vi "main(Test DQMH modules).vi"() -> ()   [LabVIEW 2018, in "Application.lvlib"] (continued)
        n826 = call "Connect to CE14.vi"("Module ID"=-1) -> ("error out"=w1953:errorcluster)  [unwired: 10 in]
        n827 = Merge Errors(w1949, w1953) -> (w1946:errorcluster)
        n828 = flat-sequence {
          tunnel: [w1959] -> w1947
          tunnel: w1946 -> [w1959]
          frame #0 {
            n829 = Wait (ms)(milliseconds to wait=u32 70) -> ()  [unwired: 1 out]
          }
        }
      }
      frame "MEAS.Read EMIC connected" {
        n830 = disable-structure shown="LOGGING==TRUE" {
          disable-tunnel: w1981 -> [w1999 _]
          frame condition #0 (active) {
            n831 = Empty String/Path?(string/path=w1999) -> (empty?=w2002:bool)
            n832 = Select(t="Quece timeout", s=w2002, f=w1999) -> (s? t:f=w1998:string)
            n833 = call "string log (SubVI).vi"("Enum"=enum16{"Init", "Log", "Read"}."Log", "state Name"=w1998) -> ()  [unwired: 8 in, 2 out]
          }
          frame condition #1 {
          }
        }
        n834 = local read "CE14  Module did it"() -> (w1967:bool[])
        n835 = for {
          N: 6 -> [_]
          tunnel: [w2005] -> w1980 mode=indexing
          tunnel: [w2004] -> w1985 mode=indexing
          i -> [w2007]
          n836 = Increment(x=w2007) -> (x+1=w2006:i32)
          n837 = Wait (ms)(milliseconds to wait=u32 50) -> ()  [unwired: 1 out]
          n838 = call "CE14.CheckConnected.vi"("Module ID"=w2006) -> ("error out"=w2004:errorcluster, "Success"=w2005:bool)  [unwired: 8 in, 1 out]
        }
        "EMIC connected" <- w1980
        n839 = And(x=w1967, y=w1980) -> (x .and. y?=w1970:bool[])
        n840 = Index Array(array=w1970) -> (element #1=→"Inst. 4":bool, element #2=→"Inst. 5":bool, element #3=→"Inst. 6":bool, element #4=→"Inst. 7":bool, element #5=→"Inst. 8":bool, element #6=→"Inst. 9":bool)  [unwired: 6 in]
        n841 = Merge Errors(w1984, w1985) -> (w1972:errorcluster)
        n842 = for {
          tunnel: w1970 -> [w1995] mode=indexing
          tunnel: [w1994] -> w1969
          n843 = call "FGV Init phase.vi"("Boolean"=w1995) -> ("Init Completed?"=w1994:bool)  [unwired: 9 in, 1 out]
        }
        n844 = case shown="False" w1969 {
          tunnel: w1968 -> [_ w1993]
          tunnel: [_ w1991] -> w1965
          frame False {
          }
          frame True {
            n845 = call "App enquece.vi"("command"="INIT.Read DRV code", "queue in"=w1993) -> ("error out"=w1991:errorcluster)  [unwired: 8 in, 1 out]
          }
        }
        n846 = Merge Errors(w1972, w1965) -> (w1966:errorcluster)
        n847 = flat-sequence {
          tunnel: [w1996] -> w1973
          tunnel: w1966 -> [w1996]
          frame #0 {
            n848 = Wait (ms)(milliseconds to wait=u32 70) -> ()  [unwired: 1 out]
          }
        }
      }
      frame "MEAS.Set DMM config" {
        n849 = disable-structure shown="LOGGING==TRUE" {
          disable-tunnel: w2011 -> [w2030 _]
          frame condition #0 (active) {
            n850 = Empty String/Path?(string/path=w2030) -> (empty?=w2033:bool)
            n851 = Select(t="Quece timeout", s=w2033, f=w2030) -> (s? t:f=w2029:string)
            n852 = call "string log (SubVI).vi"("Enum"=enum16{"Init", "Log", "Read"}."Log", "state Name"=w2029) -> ()  [unwired: 8 in, 2 out]
          }
          frame condition #1 {
          }
        }
        n853 = Variant To Data(type=T19 {"DMM config cluster"={"DCV range"=0.0, "DCI range"=0.0, "Detector Rate"=0}, "mux2-1(DMM I) encode"=enum."DMM I (0.5)"} ("DMM all config"), Variant=w2023) -> (data=w2021:T19)  [unwired: 1 in, 1 out]
        n854 = Unbundle By Name(w2021) -> ("DMM config cluster"=w2020:T20)
        n855 = Unbundle By Name(w2020) -> ("DCV range"=w2019:dbl, "DCI range"=w2018:dbl, "Detector Rate"=w2017:u8)
        n856 = call "config channel.vi"("Detector Rate"=w2017, "DCI range"=w2018, "DCV range"=w2019) -> ("error out"=w2015:errorcluster)  [unwired: 8 in]
        n857 = Merge Errors(w2012, w2015) -> (w2009:errorcluster)
        n858 = flat-sequence {
          tunnel: [w2028] -> w2010
          tunnel: w2009 -> [w2028]
          frame #0 {
            n859 = Wait (ms)(milliseconds to wait=u32 70) -> ()  [unwired: 1 out]
          }
        }
      }
      frame "MEAS.AllRelaysOFF" {
        n860 = disable-structure shown="LOGGING==TRUE" {
          disable-tunnel: w2036 -> [w2047 _]
          frame condition #0 (active) {
            n861 = Empty String/Path?(string/path=w2047) -> (empty?=w2050:bool)
            n862 = Select(t="Quece timeout", s=w2050, f=w2047) -> (s? t:f=w2046:string)
            n863 = call "string log (SubVI).vi"("Enum"=enum16{"Init", "Log", "Read"}."Log", "state Name"=w2046) -> ()  [unwired: 8 in, 2 out]
          }
          frame condition #1 {
          }
        }
        n864 = for {
          N: 5 -> [_]
          tunnel: [w2051] -> w2041 mode=indexing
          i -> [w2053]
          n865 = case shown="4" w2053 {
            tunnel: [w2057 w2058 w2059 w2060 w2061 _] -> w2051
            frame 0 {
              n866 = Initialize Array(FALSE, 6 ("dimension size")) -> (w2054:bool[])
              n867 = call "MB01_eMICs.vi"("Array"=w2054) -> ("error out"=w2057:errorcluster)  [unwired: 10 in]
            }
            frame 1 {
              n868 = call "demux1-10_chan0.vi"() -> ("error out"=w2058:errorcluster)  [unwired: 11 in]
            }
            frame 2 {
              n869 = call "SC enable OFF.vi"() -> ("error out"=w2059:errorcluster)  [unwired: 11 in]
            }
            frame 3 {
              n870 = call "mux10-1_chan0.vi"() -> ("error out"=w2060:errorcluster)  [unwired: 11 in]
            }
            frame 4 {
              n871 = call "mux6-1_chan0.vi"() -> ("error out"=w2061:errorcluster)  [unwired: 11 in]
            }
            frame 5.., Default {
            }
          }
          n872 = Wait (ms)(milliseconds to wait=u32 70) -> ()  [unwired: 1 out]
        }
        n873 = Merge Errors(w2037, w2041) -> (w2034:errorcluster)
      }
      frame "MEAS.AllRelaysOFF2" {
        # "Turn eMICs' relays OFF"
        n874 = disable-structure shown="LOGGING==TRUE" {
          disable-tunnel: w2065 -> [w2079 _]
          frame condition #0 (active) {
            n875 = Empty String/Path?(string/path=w2079) -> (empty?=w2082:bool)
            n876 = Select(t="Quece timeout", s=w2082, f=w2079) -> (s? t:f=w2078:string)
            n877 = call "string log (SubVI).vi"("Enum"=enum16{"Init", "Log", "Read"}."Log", "state Name"=w2078) -> ()  [unwired: 8 in, 2 out]
          }
          frame condition #1 {
          }
        }
        n878 = flat-sequence {
          tunnel: [w2077] -> w2063
          frame #0 {
            n879 = Initialize Array(FALSE, 6 ("dimension size")) -> (w2076:bool[])
            n880 = Wait (ms)(milliseconds to wait=u32 70) -> ()  [unwired: 1 out]
            n881 = call "MB01_eMICs.vi"("Array"=w2076) -> ("error out"=w2077:errorcluster)  [unwired: 10 in]
          }
        }
        n882 = Merge Errors(w2066, w2063) -> (w2062:errorcluster)
      }
      frame "MEAS.Read TRIGGER" {
        w2094 = T10 {"new board?"=TRUE, "new trigger"=TRUE, "last trigger"=TRUE}  # trigger infor
        # "JIG locked - rising-edge event"
        n883 = disable-structure shown="LOGGING==TRUE" {
          disable-tunnel: w2098 -> [w2112 _]
          frame condition #0 (active) {
            n884 = Empty String/Path?(string/path=w2112) -> (empty?=w2115:bool)
            n885 = Select(t="Quece timeout", s=w2115, f=w2112) -> (s? t:f=w2111:string)
            n886 = call "string log (SubVI).vi"("Enum"=enum16{"Init", "Log", "Read"}."Log", "state Name"=w2111) -> ()  [unwired: 8 in, 2 out]
          }
          frame condition #1 {
          }
        }
        n887 = call "Read JIG trigger.vi"() -> ("error out"=w2102:errorcluster, "Trigger?"=w2084:bool)  [unwired: 9 in, 1 out]
        "trigger Value" <- w2084
        n888 = feedback-in #3(w2084) -> ()
        n889 = feedback #3(FALSE) -> (w2091:bool)
        n890 = Greater?(x=w2084, y=w2091) -> (0:w2086:bool)
        n891 = Bundle By Name(cluster=w2094, "new board?"=w2086, "new trigger"=w2084, "last trigger"=w2091) -> (w2093:T10)
        n892 = local read "Auto/Man"() -> (w2083:bool)
        n893 = Select(t=-1, s=w2086, f=w2088) -> (s? t:f=w2089:i32)
        n894 = local write "New board?"(w2086) -> ()
        n895 = local write "new Trigger?"(w2084) -> ()
        n896 = local write "last Trigger?"(w2091) -> ()
        n897 = And(x=w2083, y=w2086) -> (x .and. y?=w2085:bool)
        n898 = case shown="True" w2085 {
          tunnel: w2095 -> [_ w2110]
          tunnel: w2093 -> [_ w2109]
          tunnel: [_ w2108] -> w2092
          frame False {
          }
          frame True {
            n899 = Generate User Event(user event=w2110, event data cluster=w2109) -> (error out=w2108:errorcluster)  [unwired: 2 in, 1 out]
          }
        }
        n900 = Merge Errors(w2101, w2102) -> (w2099:errorcluster)
        n901 = Merge Errors(w2099, w2092) -> (w2096:errorcluster)
        n902 = flat-sequence {
          tunnel: [w2116] -> w2100
          tunnel: w2096 -> [w2116]
          frame #0 {
            n903 = Wait (ms)(milliseconds to wait=u32 10) -> ()  [unwired: 1 out]
          }
        }
      }
      frame "MEAS.Sel Input Current" {
        n904 = disable-structure shown="LOGGING==TRUE" {
          disable-tunnel: w2119 -> [w2134 _]
          frame condition #0 (active) {
            n905 = Empty String/Path?(string/path=w2134) -> (empty?=w2137:bool)
            n906 = Select(t="Quece timeout", s=w2137, f=w2134) -> (s? t:f=w2133:string)
            n907 = call "string log (SubVI).vi"("Enum"=enum16{"Init", "Log", "Read"}."Log", "state Name"=w2133) -> ()  [unwired: 8 in, 2 out]
          }
          frame condition #1 {
          }
        }
        n908 = Variant To Data(type=enum16{"DMM I (0.5)", "DMM I (12)"}."DMM I (0.5)" ("mux2-1(DMM I) encode"), Variant=w2127) -> (data=w2126:enum16{"DMM I (0.5)", "DMM I (12)"})  [unwired: 1 in, 1 out]
        n909 = call "DMM I 0.5_10.vi"("mux2-1(DMM I) encode"=w2126) -> ("error out"=w2129:errorcluster)  [unwired: 10 in]
        n910 = Merge Errors(w2122, w2129) -> (w2120:errorcluster)
        n911 = flat-sequence {
          tunnel: [w2138] -> w2121
          tunnel: w2120 -> [w2138]
          frame #0 {
            n912 = Wait (ms)(milliseconds to wait=u32 70) -> ()  [unwired: 1 out]
          }
        }
      }
      frame "MEAS.Read Optos" {
        n913 = disable-structure shown="LOGGING==TRUE" {
          disable-tunnel: w2143 -> [w2168 _]
          frame condition #0 (active) {
            n914 = Empty String/Path?(string/path=w2168) -> (empty?=w2171:bool)
            n915 = Select(t="Quece timeout", s=w2171, f=w2168) -> (s? t:f=w2167:string)
            n916 = call "string log (SubVI).vi"("Enum"=enum16{"Init", "Log", "Read"}."Log", "state Name"=w2167) -> ()  [unwired: 8 in, 2 out]
          }
          frame condition #1 {
          }
        }
        n917 = flat-sequence {
          tunnel: [w2157] -> w2141
          frame #0 {
            n918 = disable-structure shown="Enabled" {
              frame Enabled {
                n919 = Wait (ms)(milliseconds to wait=u32 100) -> ()  [unwired: 1 out]
              }
              frame Disabled {
              }
            }
            n920 = Initialize Array(FALSE, 6 ("dimension size"), 10 ("dimension size")) -> (w2152:bool[][])
            n921 = local write "Short DRV"(w2152) -> ()
          }
          frame #1 {
            n922 = call "inst.Optos.vi"() -> ("error out"=w2166:errorcluster, "Optos"=w2164:bool[])  [unwired: 9 in, 1 out]
            n923 = Reshape Array(w2164, 10 ("dimension size"), 6 ("dimension size")) -> (w2162:bool[][])
            n924 = To Variant(anything=w2164) -> (Variant=w2165:variant)
            n925 = Transpose 2D Array(2D array=w2162) -> (transposed array=→"Short DRV":bool[][])
            n926 = call "FGV Driver Data.vi"("Mode"=DUT_data_Mode."Short Circuits", "error in (no error)"=w2166, "FGV enum(Read)"=FGV_DRV_data."Write" ("FGV DRV data enum"), "data"=w2165) -> ("error out"=w2157:errorcluster)  [unwired: 4 in, 3 out]
          }
        }
        n927 = Merge Errors(w2142, w2141) -> (w2144:errorcluster)
        n928 = flat-sequence {
          tunnel: [w2172] -> w2145
          tunnel: w2144 -> [w2172]
          frame #0 {
            n929 = Wait (ms)(milliseconds to wait=u32 70) -> ()  [unwired: 1 out]
          }
        }
      }
      frame "MEAS.Reset JIG" {
        n930 = disable-structure shown="LOGGING==TRUE" {
          disable-tunnel: w2178 -> [w2188 _]
          frame condition #0 (active) {
            n931 = Empty String/Path?(string/path=w2188) -> (empty?=w2191:bool)
            n932 = Select(t="Quece timeout", s=w2191, f=w2188) -> (s? t:f=w2187:string)
            n933 = call "string log (SubVI).vi"("Enum"=enum16{"Init", "Log", "Read"}."Log", "state Name"=w2187) -> ()  [unwired: 8 in, 2 out]
          }
          frame condition #1 {
          }
        }
        n934 = disable-structure shown="Enabled" {
          disable-tunnel: w2176 -> [w2186 _]
          frame Disabled {
            n935 = call "reset DRV UI (SubVI).vi"("Ref  in"=w2186) -> ()  [unwired: 9 in, 2 out]
          }
          frame Enabled {
          }
        }
        n936 = call "JIG Reset.vi"() -> ("error out"=w2183:errorcluster)  [unwired: 11 in]
        n937 = Merge Errors(w2179, w2183) -> (w2174:errorcluster)
      }
      frame "MEAS.Turn+5V" {
        n938 = disable-structure shown="LOGGING==TRUE" {
          disable-tunnel: w2194 -> [w2210 _]
          frame condition #0 (active) {
            n939 = Empty String/Path?(string/path=w2210) -> (empty?=w2213:bool)
            n940 = Select(t="Quece timeout", s=w2213, f=w2210) -> (s? t:f=w2209:string)
            n941 = call "string log (SubVI).vi"("Enum"=enum16{"Init", "Log", "Read"}."Log", "state Name"=w2209) -> ()  [unwired: 8 in, 2 out]
          }
          frame condition #1 {
          }
        }
        n942 = Variant To Data(type=TRUE, Variant=w2203) -> (data=w2193:bool)  [unwired: 1 in, 1 out]
        n943 = case shown="True" w2193 {
          tunnel: [w2207 w2208] -> w2200
          frame False {
            n944 = call "SC enable OFF.vi"() -> ("error out"=w2207:errorcluster)  [unwired: 11 in]
          }
          frame True {
            n945 = call "SC enable ON.vi"() -> ("error out"=w2208:errorcluster)  [unwired: 11 in]
          }
        }
        n946 = Merge Errors(w2195, w2200) -> (w2196:errorcluster)
        n947 = flat-sequence {
          tunnel: w2196 -> [w2214]
          tunnel: [w2214] -> w2199
          frame #0 {
            n948 = Wait (ms)(milliseconds to wait=u32 2000) -> ()  [unwired: 1 out]
          }
        }
      }
      frame "MEAS.demux1-10" {
        n949 = disable-structure shown="LOGGING==TRUE" {
          disable-tunnel: w2219 -> [w2248 _]
          frame condition #0 (active) {
            n950 = Empty String/Path?(string/path=w2248) -> (empty?=w2251:bool)
            n951 = Select(t="Quece timeout", s=w2251, f=w2248) -> (s? t:f=w2247:string)
            n952 = call "string log (SubVI).vi"("Enum"=enum16{"Init", "Log", "Read"}."Log", "state Name"=w2247) -> ()  [unwired: 8 in, 2 out]
          }
          frame condition #1 {
          }
        }
        n953 = Variant To Data(type=T6."demux1_10_channel0" ("demux1_10(x6)_encode"), Variant=w2227) -> (data=w2218:T6)  [unwired: 1 in, 1 out]
        n954 = case shown="\"demux1_10_channel1\"" w2218 {
          tunnel: [w2236 w2237 w2238 w2239 w2240 w2241 w2242 w2243 w2244 w2245 w2246] -> w2217
          frame "demux1_10_channel0", Default {
            n955 = call "demux1-10_chan0.vi"() -> ("error out"=w2236:errorcluster)  [unwired: 11 in]
          }
          frame "demux1_10_channel1" {
            n956 = call "demux1-10_chan1.vi"() -> ("error out"=w2237:errorcluster)  [unwired: 11 in]
          }
          frame "demux1_10_channel2" {
            n957 = call "demux1-10_chan2.vi"() -> ("error out"=w2238:errorcluster)  [unwired: 11 in]
          }
          frame "demux1_10_channel3" {
            n958 = call "demux1-10_chan3.vi"() -> ("error out"=w2239:errorcluster)  [unwired: 11 in]
          }
          frame "demux1_10_channel4" {
            n959 = call "demux1-10_chan4.vi"() -> ("error out"=w2240:errorcluster)  [unwired: 11 in]
          }
          frame "demux1_10_channel5" {
            n960 = call "demux1-10_chan5.vi"() -> ("error out"=w2241:errorcluster)  [unwired: 11 in]
          }
          frame "demux1_10_channel6" {
            n961 = call "demux1-10_chan6.vi"() -> ("error out"=w2242:errorcluster)  [unwired: 11 in]
          }
          frame "demux1_10_channel7" {
            n962 = call "demux1-10_chan7.vi"() -> ("error out"=w2243:errorcluster)  [unwired: 11 in]
          }
          frame "demux1_10_channel8" {
            n963 = call "demux1-10_chan8.vi"() -> ("error out"=w2244:errorcluster)  [unwired: 11 in]
          }
          frame "demux1_10_channel9" {
            n964 = call "demux1-10_chan9.vi"() -> ("error out"=w2245:errorcluster)  [unwired: 11 in]
          }
          frame "demux1_10_channel10" {
            n965 = call "demux1-10_chan10.vi"() -> ("error out"=w2246:errorcluster)  [unwired: 11 in]
          }
        }
        n966 = Merge Errors(w2220, w2217) -> (w2221:errorcluster)
        n967 = disable-structure shown="Enabled" {
          disable-tunnel: [w2232 w2235] -> w2222
          disable-tunnel: w2221 -> [w2231 w2235]
          frame Enabled {
            n968 = flat-sequence {
              tunnel: [w2233] -> w2232
              tunnel: w2231 -> [w2233]
              frame #0 {
                n969 = Wait (ms)(milliseconds to wait="1-10delay") -> ()  [unwired: 1 out]
              }
            }
          }
          frame Disabled {
          }
        }
      }
      frame "MEAS.eMIC" {
        # "eliminated shorted Circuits"
        n970 = disable-structure shown="LOGGING==TRUE" {
          disable-tunnel: w2254 -> [w2280 _]
          frame condition #0 (active) {
            n971 = Empty String/Path?(string/path=w2280) -> (empty?=w2283:bool)
            n972 = Select(t="Quece timeout", s=w2283, f=w2280) -> (s? t:f=w2279:string)
            n973 = call "string log (SubVI).vi"("Enum"=enum16{"Init", "Log", "Read"}."Log", "state Name"=w2279) -> ()  [unwired: 8 in, 2 out]
          }
          frame condition #1 {
          }
        }
        n974 = call "FGV Driver Data.vi"("DUT channel (1-11)"=w2256, "FGV enum(Read)"=FGV_DRV_data."Read" ("FGV DRV data enum")) -> ("Short Circuits?"=w2265:bool[])  [unwired: 6 in, 3 out]
        n975 = Variant To Data(type=bool[] [], Variant=w2270) -> (data=w2263:bool[])  [unwired: 1 in, 1 out]
        n976 = Not(x=w2265) -> (.not. x?=w2264:bool[])
        n977 = And(x=w2264, y=w2263) -> (x .and. y?=w2262:bool[])
        n978 = call "MB01_eMICs.vi"("Array"=w2262) -> ("error out"=w2260:errorcluster)  [unwired: 10 in]
        n979 = call "FGV wait for 6 eMICs.vi"("Enum"=enum16{"Init", "count"}."Init", "error in (no error)"=w2260) -> ("error out"=w2252:errorcluster, "wait done"=w2261:bool)  [unwired: 7 in, 1 out]
        n980 = Merge Errors(w2255, w2252) -> (w2257:errorcluster)
        n981 = local write "AC  Completed"(w2261) -> ()
        n982 = disable-structure shown="Enabled" {
          disable-tunnel: [w2275 w2278] -> w2258
          disable-tunnel: w2257 -> [w2274 w2278]
          frame Enabled {
            n983 = flat-sequence {
              tunnel: [w2277] -> w2275
              tunnel: w2274 -> [w2277]
              frame #0 {
                n984 = Wait (ms)(milliseconds to wait="eMIC delay") -> ()  [unwired: 1 out]
              }
            }
          }
          frame Disabled {
          }
        }
      }
      frame "MEAS.requestAC" {
        n985 = disable-structure shown="LOGGING==TRUE" {
          disable-tunnel: w2287 -> [w2316 _]
          frame condition #0 (active) {
            n986 = Empty String/Path?(string/path=w2316) -> (empty?=w2319:bool)
            n987 = Select(t="Quece timeout", s=w2319, f=w2316) -> (s? t:f=w2315:string)
            n988 = call "string log (SubVI).vi"("Enum"=enum16{"Init", "Log", "Read"}."Log", "state Name"=w2315) -> ()  [unwired: 8 in, 2 out]
          }
          frame condition #1 {
          }
        }
        n989 = Variant To Data(type=-1 ("Module ID"), Variant=w2285) -> (data=w2284:i32)  [unwired: 1 in, 1 out]
        n990 = case shown="0" w2284 {
          selector: w2284 -> [w2304 _]
          tunnel: [w2303 w2308] -> w2291
          frame 1, Default {
            n991 = Quotient & Remainder(x=w2304, y=6) -> (x-y*floor(x/y)=w2300:i32)  [unwired: 1 out]
            n992 = Equal To 0?(x=w2300) -> (x = 0?=w2302:bool)
            n993 = Select(t=6, s=w2302, f=w2300) -> (s? t:f=w2299:i32)
            n994 = call "Read AC parameters.vi"("Module ID"=w2299) -> ("error out"=w2303:errorcluster)  [unwired: 10 in]
          }
          frame 0 {
            n995 = call "FGV wait for 6 eMICs.vi"("Enum"=enum16{"Init", "count"}."Init") -> ("error out"=w2306:errorcluster)  [unwired: 8 in, 2 out]
            n996 = call "Read AC parameters.vi"("error in"=w2306, "Module ID"=-1) -> ("error out"=w2308:errorcluster)  [unwired: 9 in]
          }
        }
        n997 = Merge Errors(w2292, w2291) -> (w2289:errorcluster)
        n998 = disable-structure shown="Enabled" {
          disable-tunnel: [w2311 w2314] -> w2290
          disable-tunnel: w2289 -> [w2310 w2314]
          frame Disabled {
            n999 = flat-sequence {
              tunnel: [w2312] -> w2311
              tunnel: w2310 -> [w2312]
              frame #0 {
                n1000 = Wait (ms)(milliseconds to wait=u32 70) -> ()  [unwired: 1 out]
              }
            }
          }
          frame Enabled {
          }
        }
      }
      frame "MEAS.mux6_1" {
        n1001 = disable-structure shown="LOGGING==TRUE" {
          disable-tunnel: w2326 -> [w2369 _]
          frame condition #0 (active) {
            n1002 = Empty String/Path?(string/path=w2369) -> (empty?=w2372:bool)
            n1003 = Select(t="Quece timeout", s=w2372, f=w2369) -> (s? t:f=w2368:string)
            n1004 = call "string log (SubVI).vi"("Enum"=enum16{"Init", "Log", "Read"}."Log", "state Name"=w2368) -> ()  [unwired: 8 in, 2 out]
          }
          frame condition #1 {
          }
        }
        n1005 = Variant To Data(type=T4."mux6-1_channel0" ("mux6_1(3wires)_encode"), Variant=w2334) -> (data=w2325:T4)  [unwired: 1 in, 1 out]
        n1006 = case shown="\"mux6_1_channel6_3\"" w2325 {
          tunnel: [w2343 w2345 w2347 w2349 w2351 w2353 w2355 w2357 w2359 w2361 w2363 w2365 w2367] -> w2324
          tunnel: [w2342 w2344 w2346 w2348 w2350 w2352 w2354 w2356 w2358 w2360 w2362 w2364 w2366] -> w2320
          tunnel: "6_1 delay" -> [_ _ w2346 _ w2350 _ w2354 _ w2358 _ w2362 _ w2366]
          tunnel: "6_1 delay2" -> [w2342 w2344 _ w2348 _ w2352 _ w2356 _ w2360 _ w2364 _]
          frame "mux6-1_channel0", Default {
            n1007 = call "mux6-1_chan0.vi"() -> ("error out"=w2343:errorcluster)  [unwired: 11 in]
          }
          frame "mux6-1_channel1_2" {
            n1008 = call "mux6-1_chan1_1.vi"() -> ("error out"=w2345:errorcluster)  [unwired: 11 in]
          }
          frame "mux6_1_channel1_3" {
            n1009 = call "mux6-1_chan1_2.vi"() -> ("error out"=w2347:errorcluster)  [unwired: 11 in]
          }
          frame "mux6_1_channel2_2" {
            n1010 = call "mux6-1_chan2_1.vi"() -> ("error out"=w2349:errorcluster)  [unwired: 11 in]
          }
          frame "mux6_1_channel2_3" {
            n1011 = call "mux6-1_chan2_2.vi"() -> ("error out"=w2351:errorcluster)  [unwired: 11 in]
          }
          frame "mux6_1_channel3_2" {
            n1012 = call "mux6-1_chan3_1.vi"() -> ("error out"=w2353:errorcluster)  [unwired: 11 in]
          }
          frame "mux6_1_channel3_3" {
            n1013 = call "mux6-1_chan3_2.vi"() -> ("error out"=w2355:errorcluster)  [unwired: 11 in]
          }
          frame "mux6_1_channel4_2" {
            n1014 = call "mux6-1_chan4_1.vi"() -> ("error out"=w2357:errorcluster)  [unwired: 11 in]
          }
          frame "mux6_1_channel4_3" {
            n1015 = call "mux6-1_chan4_2.vi"() -> ("error out"=w2359:errorcluster)  [unwired: 11 in]
          }
          frame "mux6_1_channel5_2" {
            n1016 = call "mux6-1_chan5_1.vi"() -> ("error out"=w2361:errorcluster)  [unwired: 11 in]
          }
          frame "mux6_1_channel5_3" {
            n1017 = call "mux6-1_chan5_2.vi"() -> ("error out"=w2363:errorcluster)  [unwired: 11 in]
          }
          frame "mux6_1_channel6_2" {
            n1018 = call "mux6-1_chan6_1.vi"() -> ("error out"=w2365:errorcluster)  [unwired: 11 in]
          }
          frame "mux6_1_channel6_3" {
            n1019 = call "mux6-1_chan6_2.vi"() -> ("error out"=w2367:errorcluster)  [unwired: 11 in]
          }
        }
        n1020 = Merge Errors(w2329, w2324) -> (w2327:errorcluster)
        n1021 = Wait (ms)(milliseconds to wait=w2320) -> ()  [unwired: 1 out]
        n1022 = disable-structure shown="Enabled" {
          disable-tunnel: [w2339 w2341] -> w2328
          disable-tunnel: w2327 -> [w2338 w2341]
          frame Enabled {
            n1023 = flat-sequence {
              tunnel: [w2340] -> w2339
              tunnel: w2338 -> [w2340]
              frame #0 {
              }
            }
          }
          frame Disabled {
          }
        }
      }
      frame "MEAS.mux10-1" {
        n1024 = disable-structure shown="LOGGING==TRUE" {
          disable-tunnel: w2376 -> [w2405 _]
          frame condition #0 (active) {
            n1025 = Empty String/Path?(string/path=w2405) -> (empty?=w2408:bool)
            n1026 = Select(t="Quece timeout", s=w2408, f=w2405) -> (s? t:f=w2404:string)
            n1027 = call "string log (SubVI).vi"("Enum"=enum16{"Init", "Log", "Read"}."Log", "state Name"=w2404) -> ()  [unwired: 8 in, 2 out]
          }
          frame condition #1 {
          }
        }
        n1028 = Variant To Data(type=T5."mux10_1_channel0" ("mux10_1(x6)_encode"), Variant=w2384) -> (data=w2375:T5)  [unwired: 1 in, 1 out]
        n1029 = case shown="\"mux10_1_channel1\"" w2375 {
          tunnel: [w2393 w2394 w2395 w2396 w2397 w2398 w2399 w2400 w2401 w2402 w2403] -> w2374
          frame "mux10_1_channel0", Default {
            n1030 = call "mux10-1_chan0.vi"() -> ("error out"=w2393:errorcluster)  [unwired: 11 in]
          }
          frame "mux10_1_channel1" {
            n1031 = call "mux10-1_chan1.vi"() -> ("error out"=w2394:errorcluster)  [unwired: 11 in]
          }
          frame "mux10_1_channel2" {
            n1032 = call "mux10-1_chan2.vi"() -> ("error out"=w2395:errorcluster)  [unwired: 11 in]
          }
          frame "mux10_1_channel3" {
            n1033 = call "mux10-1_chan3.vi"() -> ("error out"=w2396:errorcluster)  [unwired: 11 in]
          }
          frame "mux10_1_channel4" {
            n1034 = call "mux10-1_chan4.vi"() -> ("error out"=w2397:errorcluster)  [unwired: 11 in]
          }
          frame "mux10_1_channel5" {
            n1035 = call "mux10-1_chan5.vi"() -> ("error out"=w2398:errorcluster)  [unwired: 11 in]
          }
          frame "mux10_1_channel6" {
            n1036 = call "mux10-1_chan6.vi"() -> ("error out"=w2399:errorcluster)  [unwired: 11 in]
          }
          frame "mux10_1_channel7" {
            n1037 = call "mux10-1_chan7.vi"() -> ("error out"=w2400:errorcluster)  [unwired: 11 in]
          }
          frame "mux10_1_channel8" {
            n1038 = call "mux10-1_chan8.vi"() -> ("error out"=w2401:errorcluster)  [unwired: 11 in]
          }
          frame "mux10_1_channel9" {
            n1039 = call "mux10-1_chan9.vi"() -> ("error out"=w2402:errorcluster)  [unwired: 11 in]
          }
          frame "mux10_1_channel10" {
            n1040 = call "mux10-1_chan10.vi"() -> ("error out"=w2403:errorcluster)  [unwired: 11 in]
          }
        }
        n1041 = Merge Errors(w2379, w2374) -> (w2378:errorcluster)
        n1042 = disable-structure shown="Enabled" {
          disable-tunnel: w2378 -> [w2389 w2392]
          disable-tunnel: [w2388 w2392] -> w2377
          frame Enabled {
            n1043 = flat-sequence {
              tunnel: w2389 -> [w2390]
              tunnel: [w2390] -> w2388
              frame #0 {
                n1044 = Wait (ms)(milliseconds to wait="10-1 delay") -> ()  [unwired: 1 out]
              }
            }
          }
          frame Disabled {
          }
        }
      }
      frame "MEAS.DMM dual read" {
        n1045 = disable-structure shown="LOGGING==TRUE" {
          disable-tunnel: w2416 -> [w2442 _]
          frame condition #0 (active) {
            n1046 = Empty String/Path?(string/path=w2442) -> (empty?=w2445:bool)
            n1047 = Select(t="Quece timeout", s=w2445, f=w2442) -> (s? t:f=w2441:string)
            n1048 = call "string log (SubVI).vi"("Enum"=enum16{"Init", "Log", "Read"}."Log", "state Name"=w2441) -> ()  [unwired: 8 in, 2 out]
          }
          frame condition #1 {
          }
        }
        n1049 = call "FGV Driver Data.vi"("DUT index(1-60)"=w2409) -> ("DUT SC"=w2410:bool)  [unwired: 7 in, 3 out]
        n1050 = case shown="False" w2410 {
          tunnel: [w2423 _] -> w2412
          tunnel: w2409 -> [w2424 _]
          frame False {
            n1051 = flat-sequence {
              tunnel: [w2427] -> w2425
              tunnel: w2424 -> [w2427]
              tunnel: w2425 -> [w2430]
              tunnel: [w2429] -> w2423
              frame #0 {
                w2426 = 0.0 ("DCV(Volts)")
                n1052 = disable-structure shown="Enabled" {
                  frame Enabled {
                    n1053 = Wait (ms)(milliseconds to wait=u32 50) -> ()  [unwired: 1 out]
                  }
                  frame Disabled {
                  }
                }
                n1054 = local write "DCV(Volts)"(w2426) -> ()
                n1055 = local write "DCI(mA)"(w2426) -> ()
              }
              frame #1 {
                w2431 = u16 2 items=["1st Display", "2nd Display", "1st & 2nd Display"] ("Sets to Display")
                n1056 = call "Read DCV_DCI.vi"("Sets to Display"=w2431) -> ("error out"=w2434:errorcluster, "DCI"=w2438:dbl, "DCV"=w2437:dbl)  [unwired: 7 in, 1 out]
                "DCI(mA)" <- w2438
                "DCV(Volts)" <- w2437
                n1057 = Build Array(w2437, w2438) -> (w2436:dbl[])
                n1058 = To Variant(anything=w2436) -> (Variant=w2435:variant)
                n1059 = call "FGV Driver Data.vi"("Mode"=DUT_data_Mode."DC parameter", "DUT index(1-60)"=w2430, "error in (no error)"=w2434, "FGV enum(Read)"=FGV_DRV_data."Write" ("FGV DRV data enum"), "data"=w2435) -> ("error out"=w2429:errorcluster)  [unwired: 3 in, 3 out]
              }
            }
          }
          frame True {
          }
        }
        n1060 = Merge Errors(w2417, w2412) -> (w2414:errorcluster)
        n1061 = flat-sequence {
          tunnel: [w2440] -> w2415
          tunnel: w2414 -> [w2440]
          frame #0 {
            n1062 = Wait (ms)(milliseconds to wait="DMM delay") -> ()  [unwired: 1 out]
          }
        }
      }
      frame "Test Shorted Circuits" {
        w2452 = T25 {"command"="", "Data"=variant} ("Variant")
        n1063 = disable-structure shown="LOGGING==TRUE" {
          disable-tunnel: w2461 -> [w2481 _]
          frame condition #0 (active) {
            n1064 = Empty String/Path?(string/path=w2481) -> (empty?=w2484:bool)
            n1065 = Select(t="Quece timeout", s=w2484, f=w2481) -> (s? t:f=w2480:string)
            n1066 = call "string log (SubVI).vi"("Enum"=enum16{"Init", "Log", "Read"}."Log", "state Name"=w2480) -> ()  [unwired: 8 in, 2 out]
          }
          frame condition #1 {
          }
        }
        n1067 = To Variant(anything=TRUE) -> (Variant=w2471:variant)
        n1068 = To Variant(anything=FALSE) -> (Variant=w2456:variant)
        n1069 = Bundle By Name(cluster=w2452, "command"="MEAS.AllRelaysOFF") -> (w2473:T25)
        n1070 = Bundle By Name(cluster=w2452, "command"="MEAS.Turn+5V", "Data"=w2471) -> (w2472:T25)
        n1071 = Bundle By Name(cluster=w2452, "command"="MEAS.Read Optos") -> (w2469:T25)
        n1072 = Bundle By Name(cluster=w2452, "command"="MEAS.Turn+5V", "Data"=w2456) -> (w2460:T25)
        n1073 = Bundle By Name(cluster=w2452, "command"="Apps.UI Update SC") -> (w2450:T25)
        n1074 = Build Array(w2473, w2472, w2469, w2460, w2450) -> (w2462:T25[])
        n1075 = Reverse 1D Array(array=w2462) -> (reversed array=w2463:T25[])
        n1076 = for {
          tunnel: w2463 -> [w2488] mode=indexing
          tunnel: w2467 -> [w2490]
          tunnel: [w2489] -> w2454 mode=indexing
          n1077 = Unbundle By Name(w2488) -> ("command"=w2487:string, "Data"=w2486:variant)
          n1078 = call "App enquece.vi"("Priority Enquece"=TRUE, "command data"=w2486, "command"=w2487, "queue in"=w2490) -> ("error out"=w2489:errorcluster)  [unwired: 6 in, 1 out]
        }
        n1079 = call "reset DRV UI (SubVI).vi"("Ref  in"=w2466) -> ("error out"=w2447:errorcluster)  [unwired: 9 in, 1 out]
        n1080 = call "FGV Driver Data.vi"("error in (no error)"=w2447, "FGV enum(Read)"=FGV_DRV_data."Init" ("FGV DRV data enum")) -> ("error out"=w2446:errorcluster)  [unwired: 6 in, 3 out]
        n1081 = Merge Errors(w2455, w2454) -> (w2459:errorcluster)
        n1082 = Merge Errors(w2459, w2446) -> (w2449:errorcluster)
      }
      frame "Test Channel 1" {
        w2520 = 1  # DUT channel (1-11)
        w2521 = T11 {"command"="", "command data"=variant} ("element")
        n1083 = disable-structure shown="LOGGING==TRUE" {
          disable-tunnel: w2516 -> [w2551 _]
          frame condition #0 (active) {
            n1084 = Empty String/Path?(string/path=w2551) -> (empty?=w2554:bool)
            n1085 = Select(t="Quece timeout", s=w2554, f=w2551) -> (s? t:f=w2550:string)
            n1086 = call "string log (SubVI).vi"("Enum"=enum16{"Init", "Log", "Read"}."Log", "state Name"=w2550) -> ()  [unwired: 8 in, 2 out]
          }
          frame condition #1 {
          }
        }
        n1087 = Build Array("Apps.UI Update", "MEAS.AllRelaysOFF2", "Apps.WaitForEvent") -> (w2500:string[])
        n1088 = for {
          tunnel: [w2541] -> w2502 mode=indexing
          shift-right: [w2540] -> w2501
          shift-left: w2503 -> [w2543]
          tunnel: w2500 -> [w2539] mode=indexing
          n1089 = call "App enquece.vi"("Priority Enquece"=TRUE, "command"=w2539, "queue in"=w2543) -> ("error out"=w2541:errorcluster, "Queue out"=w2540:refnum<queue>)  [unwired: 7 in]
        }
        n1090 = Build Array("Test DRV 1", "Test DRV 2", "Test DRV 3", "Test DRV 4", "Test DRV 5", "Test DRV 6", "MEAS.requestAC") -> (w2513:string[])
        n1091 = Merge Errors(w2502) -> (w2497:errorcluster)
        n1092 = Reverse 1D Array(array=w2513) -> (reversed array=w2514:string[])
        n1093 = for {
          tunnel: w2514 -> [w2548] mode=indexing
          tunnel: [w2547] -> w2507 mode=indexing
          shift-right: [w2546] -> w2508
          shift-left: w2501 -> [w2549]
          tunnel: w2497 -> [w2545]
          n1094 = call "App enquece.vi"("Priority Enquece"=TRUE, "error in (no error)"=w2545, "command"=w2548, "queue in"=w2549) -> ("error out"=w2547:errorcluster, "Queue out"=w2546:refnum<queue>)  [unwired: 6 in]
        }
        n1095 = Initialize Array(TRUE, 6 ("dimension size")) -> (w2524:bool[])
        n1096 = To Variant(anything=w2524) -> (Variant=w2523:variant)
        n1097 = To Variant(anything=T6."demux1_10_channel1" ("demux1_10(x6)_encode")) -> (Variant=w2530:variant)
        n1098 = To Variant(anything=T5."mux10_1_channel1" ("mux10_1(x6)_encode")) -> (Variant=w2534:variant)
        n1099 = Bundle By Name(cluster=w2521, "command"="MEAS.mux10-1", "command data"=w2534) -> (w2529:T11)
        n1100 = Bundle By Name(cluster=w2521, "command"="MEAS.demux1-10", "command data"=w2530) -> (w2528:T11)
        n1101 = Bundle By Name(cluster=w2521, "command"="MEAS.eMIC", "command data"=w2523) -> (w2522:T11)
        n1102 = Build Array(w2529, w2528, w2522) -> (w2505:T11[])
        n1103 = Merge Errors(w2507) -> (w2506:errorcluster)
        n1104 = Reverse 1D Array(array=w2505) -> (reversed array=w2504:T11[])
        n1105 = for {
          tunnel: w2504 -> [w2560] mode=indexing
          tunnel: [w2557] -> w2515 mode=indexing
          tunnel: w2506 -> [w2556]
          tunnel: w2508 -> [w2561]
          n1106 = Unbundle By Name(w2560) -> ("command"=w2559:string, "command data"=w2558:variant)
          n1107 = call "App enquece.vi"("Priority Enquece"=TRUE, "error in (no error)"=w2556, "command data"=w2558, "command"=w2559, "queue in"=w2561) -> ("error out"=w2557:errorcluster)  [unwired: 5 in, 1 out]
        }
        n1108 = Merge Errors(w2518, w2515) -> (w2519:errorcluster)
      }
      frame "Test Channel 2" {
        w2593 = 2  # DUT channel (1-11)
        w2594 = T11 {"command"="", "command data"=variant} ("element")
        n1109 = disable-structure shown="LOGGING==TRUE" {
          disable-tunnel: w2588 -> [w2622 _]
          frame condition #0 (active) {
            n1110 = Empty String/Path?(string/path=w2622) -> (empty?=w2625:bool)
            n1111 = Select(t="Quece timeout", s=w2625, f=w2622) -> (s? t:f=w2621:string)
            n1112 = call "string log (SubVI).vi"("Enum"=enum16{"Init", "Log", "Read"}."Log", "state Name"=w2621) -> ()  [unwired: 8 in, 2 out]
          }
          frame condition #1 {
          }
        }
        n1113 = Build Array("Apps.UI Update", "MEAS.AllRelaysOFF2", "Apps.WaitForEvent") -> (w2567:string[])
        n1114 = for {
          tunnel: [w2613] -> w2578 mode=indexing
          shift-right: [w2614] -> w2580
          shift-left: w2573 -> [w2612]
          tunnel: w2567 -> [w2610] mode=indexing
          n1115 = call "App enquece.vi"("Priority Enquece"=TRUE, "command"=w2610, "queue in"=w2612) -> ("error out"=w2613:errorcluster, "Queue out"=w2614:refnum<queue>)  [unwired: 7 in]
        }
        n1116 = Merge Errors(w2578) -> (w2570:errorcluster)
        n1117 = Build Array("Test DRV 7", "Test DRV 8", "Test DRV 9", "Test DRV 10", "Test DRV 11", "Test DRV 12", "MEAS.requestAC") -> (w2585:string[])
        n1118 = Reverse 1D Array(array=w2585) -> (reversed array=w2586:string[])
        n1119 = for {
          tunnel: w2586 -> [w2615] mode=indexing
          tunnel: [w2619] -> w2577 mode=indexing
          shift-right: [w2618] -> w2579
          shift-left: w2580 -> [w2620]
          tunnel: w2570 -> [w2617]
          n1120 = call "App enquece.vi"("Priority Enquece"=TRUE, "error in (no error)"=w2617, "command"=w2615, "queue in"=w2620) -> ("error out"=w2619:errorcluster, "Queue out"=w2618:refnum<queue>)  [unwired: 6 in]
        }
        n1121 = Initialize Array(TRUE, 6 ("dimension size")) -> (w2597:bool[])
        n1122 = To Variant(anything=T5."mux10_1_channel2" ("mux10_1(x6)_encode")) -> (Variant=w2605:variant)
        n1123 = To Variant(anything=T6."demux1_10_channel2" ("demux1_10(x6)_encode")) -> (Variant=w2602:variant)
        n1124 = To Variant(anything=w2597) -> (Variant=w2596:variant)
        n1125 = Bundle By Name(cluster=w2594, "command"="MEAS.mux10-1", "command data"=w2605) -> (w2601:T11)
        n1126 = Bundle By Name(cluster=w2594, "command"="MEAS.demux1-10", "command data"=w2602) -> (w2600:T11)
        n1127 = Bundle By Name(cluster=w2594, "command"="MEAS.eMIC", "command data"=w2596) -> (w2595:T11)
        n1128 = Merge Errors(w2577) -> (w2576:errorcluster)
        n1129 = Build Array(w2601, w2600, w2595) -> (w2575:T11[])
        n1130 = Reverse 1D Array(array=w2575) -> (reversed array=w2574:T11[])
        n1131 = for {
          tunnel: w2574 -> [w2631] mode=indexing
          tunnel: [w2628] -> w2587 mode=indexing
          tunnel: w2576 -> [w2627]
          tunnel: w2579 -> [w2632]
          n1132 = Unbundle By Name(w2631) -> ("command"=w2630:string, "command data"=w2629:variant)
          n1133 = call "App enquece.vi"("Priority Enquece"=TRUE, "error in (no error)"=w2627, "command data"=w2629, "command"=w2630, "queue in"=w2632) -> ("error out"=w2628:errorcluster)  [unwired: 5 in, 1 out]
        }
        n1134 = Merge Errors(w2590, w2587) -> (w2591:errorcluster)
      }
      frame "Test Channel 3" {
        w2663 = 3  # DUT channel (1-11)
        w2664 = T11 {"command"="", "command data"=variant} ("element")
        n1135 = disable-structure shown="LOGGING==TRUE" {
          disable-tunnel: w2658 -> [w2693 _]
          frame condition #0 (active) {
            n1136 = Empty String/Path?(string/path=w2693) -> (empty?=w2696:bool)
            n1137 = Select(t="Quece timeout", s=w2696, f=w2693) -> (s? t:f=w2692:string)
            n1138 = call "string log (SubVI).vi"("Enum"=enum16{"Init", "Log", "Read"}."Log", "state Name"=w2692) -> ()  [unwired: 8 in, 2 out]
          }
          frame condition #1 {
          }
        }
        n1139 = Build Array("Apps.UI Update", "MEAS.AllRelaysOFF2", "Apps.WaitForEvent") -> (w2641:string[])
        n1140 = for {
          tunnel: [w2683] -> w2648 mode=indexing
          shift-right: [w2684] -> w2650
          shift-left: w2644 -> [w2682]
          tunnel: w2641 -> [w2681] mode=indexing
          n1141 = call "App enquece.vi"("Priority Enquece"=TRUE, "command"=w2681, "queue in"=w2682) -> ("error out"=w2683:errorcluster, "Queue out"=w2684:refnum<queue>)  [unwired: 7 in]
        }
        n1142 = Merge Errors(w2648) -> (w2640:errorcluster)
        n1143 = Build Array("Test DRV 13", "Test DRV 14", "Test DRV 15", "Test DRV 16", "Test DRV 17", "Test DRV 18", "MEAS.requestAC") -> (w2655:string[])
        n1144 = Reverse 1D Array(array=w2655) -> (reversed array=w2656:string[])
        n1145 = for {
          tunnel: w2656 -> [w2690] mode=indexing
          tunnel: [w2689] -> w2635 mode=indexing
          shift-right: [w2688] -> w2649
          shift-left: w2650 -> [w2691]
          tunnel: w2640 -> [w2687]
          n1146 = call "App enquece.vi"("Priority Enquece"=TRUE, "error in (no error)"=w2687, "command"=w2690, "queue in"=w2691) -> ("error out"=w2689:errorcluster, "Queue out"=w2688:refnum<queue>)  [unwired: 6 in]
        }
        n1147 = Merge Errors(w2635) -> (w2647:errorcluster)
        n1148 = Initialize Array(TRUE, 6 ("dimension size")) -> (w2667:bool[])
        n1149 = To Variant(anything=T5."mux10_1_channel3" ("mux10_1(x6)_encode")) -> (Variant=w2676:variant)
        n1150 = To Variant(anything=T6."demux1_10_channel3" ("demux1_10(x6)_encode")) -> (Variant=w2672:variant)
        n1151 = To Variant(anything=w2667) -> (Variant=w2666:variant)
        n1152 = Bundle By Name(cluster=w2664, "command"="MEAS.mux10-1", "command data"=w2676) -> (w2671:T11)
        n1153 = Bundle By Name(cluster=w2664, "command"="MEAS.demux1-10", "command data"=w2672) -> (w2670:T11)
        n1154 = Bundle By Name(cluster=w2664, "command"="MEAS.eMIC", "command data"=w2666) -> (w2665:T11)
        n1155 = Build Array(w2671, w2670, w2665) -> (w2646:T11[])
        n1156 = Reverse 1D Array(array=w2646) -> (reversed array=w2645:T11[])
        n1157 = for {
          tunnel: w2645 -> [w2702] mode=indexing
          tunnel: [w2699] -> w2657 mode=indexing
          tunnel: w2647 -> [w2698]
          tunnel: w2649 -> [w2703]
          n1158 = Unbundle By Name(w2702) -> ("command"=w2701:string, "command data"=w2700:variant)
          n1159 = call "App enquece.vi"("Priority Enquece"=TRUE, "error in (no error)"=w2698, "command data"=w2700, "command"=w2701, "queue in"=w2703) -> ("error out"=w2699:errorcluster)  [unwired: 5 in, 1 out]
        }
        n1160 = Merge Errors(w2660, w2657) -> (w2661:errorcluster)
      }
      frame "Test Channel 4" {
        w2734 = 4  # DUT channel (1-11)
        w2735 = T11 {"command"="", "command data"=variant} ("element")
        n1161 = disable-structure shown="LOGGING==TRUE" {
          disable-tunnel: w2729 -> [w2764 _]
          frame condition #0 (active) {
            n1162 = Empty String/Path?(string/path=w2764) -> (empty?=w2767:bool)
            n1163 = Select(t="Quece timeout", s=w2767, f=w2764) -> (s? t:f=w2763:string)
            n1164 = call "string log (SubVI).vi"("Enum"=enum16{"Init", "Log", "Read"}."Log", "state Name"=w2763) -> ()  [unwired: 8 in, 2 out]
          }
          frame condition #1 {
          }
        }
        n1165 = Build Array("Apps.UI Update", "MEAS.AllRelaysOFF2", "Apps.WaitForEvent") -> (w2711:string[])
        n1166 = for {
          tunnel: [w2754] -> w2719 mode=indexing
          shift-right: [w2755] -> w2721
          shift-left: w2714 -> [w2753]
          tunnel: w2711 -> [w2752] mode=indexing
          n1167 = call "App enquece.vi"("Priority Enquece"=TRUE, "command"=w2752, "queue in"=w2753) -> ("error out"=w2754:errorcluster, "Queue out"=w2755:refnum<queue>)  [unwired: 7 in]
        }
        n1168 = Merge Errors(w2719) -> (w2710:errorcluster)
        n1169 = Build Array("Test DRV 19", "Test DRV 20", "Test DRV 21", "Test DRV 22", "Test DRV 23", "Test DRV 24", "MEAS.requestAC") -> (w2726:string[])
        n1170 = Reverse 1D Array(array=w2726) -> (reversed array=w2727:string[])
        n1171 = for {
          tunnel: w2727 -> [w2761] mode=indexing
          tunnel: [w2760] -> w2718 mode=indexing
          shift-right: [w2759] -> w2720
          shift-left: w2721 -> [w2762]
          tunnel: w2710 -> [w2758]
          n1172 = call "App enquece.vi"("Priority Enquece"=TRUE, "error in (no error)"=w2758, "command"=w2761, "queue in"=w2762) -> ("error out"=w2760:errorcluster, "Queue out"=w2759:refnum<queue>)  [unwired: 6 in]
        }
        n1173 = Merge Errors(w2718) -> (w2717:errorcluster)
        n1174 = Initialize Array(TRUE, 6 ("dimension size")) -> (w2738:bool[])
        n1175 = To Variant(anything=T5."mux10_1_channel4" ("mux10_1(x6)_encode")) -> (Variant=w2747:variant)
        n1176 = To Variant(anything=T6."demux1_10_channel4" ("demux1_10(x6)_encode")) -> (Variant=w2743:variant)
        n1177 = To Variant(anything=w2738) -> (Variant=w2737:variant)
        n1178 = Bundle By Name(cluster=w2735, "command"="MEAS.mux10-1", "command data"=w2747) -> (w2742:T11)
        n1179 = Bundle By Name(cluster=w2735, "command"="MEAS.demux1-10", "command data"=w2743) -> (w2741:T11)
        n1180 = Bundle By Name(cluster=w2735, "command"="MEAS.eMIC", "command data"=w2737) -> (w2736:T11)
        n1181 = Build Array(w2742, w2741, w2736) -> (w2716:T11[])
        n1182 = Reverse 1D Array(array=w2716) -> (reversed array=w2715:T11[])
        n1183 = for {
          tunnel: w2715 -> [w2773] mode=indexing
          tunnel: [w2770] -> w2728 mode=indexing
          tunnel: w2717 -> [w2769]
          tunnel: w2720 -> [w2774]
          n1184 = Unbundle By Name(w2773) -> ("command"=w2772:string, "command data"=w2771:variant)
          n1185 = call "App enquece.vi"("Priority Enquece"=TRUE, "error in (no error)"=w2769, "command data"=w2771, "command"=w2772, "queue in"=w2774) -> ("error out"=w2770:errorcluster)  [unwired: 5 in, 1 out]
        }
        n1186 = Merge Errors(w2731, w2728) -> (w2732:errorcluster)
      }
      frame "Test Channel 5" {
        w2805 = 5  # DUT channel (1-11)
        w2806 = T11 {"command"="", "command data"=variant} ("element")
        n1187 = disable-structure shown="LOGGING==TRUE" {
          disable-tunnel: w2800 -> [w2835 _]
          frame condition #0 (active) {
            n1188 = Empty String/Path?(string/path=w2835) -> (empty?=w2838:bool)
            n1189 = Select(t="Quece timeout", s=w2838, f=w2835) -> (s? t:f=w2834:string)
            n1190 = call "string log (SubVI).vi"("Enum"=enum16{"Init", "Log", "Read"}."Log", "state Name"=w2834) -> ()  [unwired: 8 in, 2 out]
          }
          frame condition #1 {
          }
        }
        n1191 = Build Array("Apps.UI Update", "MEAS.AllRelaysOFF2", "Apps.WaitForEvent") -> (w2783:string[])
        n1192 = for {
          tunnel: [w2825] -> w2791 mode=indexing
          shift-right: [w2826] -> w2792
          shift-left: w2786 -> [w2824]
          tunnel: w2783 -> [w2823] mode=indexing
          n1193 = call "App enquece.vi"("Priority Enquece"=TRUE, "command"=w2823, "queue in"=w2824) -> ("error out"=w2825:errorcluster, "Queue out"=w2826:refnum<queue>)  [unwired: 7 in]
        }
        n1194 = Merge Errors(w2791) -> (w2782:errorcluster)
        n1195 = Build Array("Test DRV 25", "Test DRV 26", "Test DRV 27", "Test DRV 28", "Test DRV 29", "Test DRV 30", "MEAS.requestAC") -> (w2797:string[])
        n1196 = Reverse 1D Array(array=w2797) -> (reversed array=w2798:string[])
        n1197 = for {
          tunnel: w2798 -> [w2832] mode=indexing
          tunnel: [w2831] -> w2790 mode=indexing
          shift-right: [w2830] -> w2781
          shift-left: w2792 -> [w2833]
          tunnel: w2782 -> [w2829]
          n1198 = call "App enquece.vi"("Priority Enquece"=TRUE, "error in (no error)"=w2829, "command"=w2832, "queue in"=w2833) -> ("error out"=w2831:errorcluster, "Queue out"=w2830:refnum<queue>)  [unwired: 6 in]
        }
        n1199 = Initialize Array(TRUE, 6 ("dimension size")) -> (w2809:bool[])
        n1200 = Merge Errors(w2790) -> (w2789:errorcluster)
        n1201 = To Variant(anything=T5."mux10_1_channel5" ("mux10_1(x6)_encode")) -> (Variant=w2818:variant)
        n1202 = To Variant(anything=T6."demux1_10_channel5" ("demux1_10(x6)_encode")) -> (Variant=w2814:variant)
        n1203 = To Variant(anything=w2809) -> (Variant=w2808:variant)
        n1204 = Bundle By Name(cluster=w2806, "command"="MEAS.mux10-1", "command data"=w2818) -> (w2813:T11)
        n1205 = Bundle By Name(cluster=w2806, "command"="MEAS.demux1-10", "command data"=w2814) -> (w2812:T11)
        n1206 = Bundle By Name(cluster=w2806, "command"="MEAS.eMIC", "command data"=w2808) -> (w2807:T11)
        n1207 = Build Array(w2813, w2812, w2807) -> (w2788:T11[])
        n1208 = Reverse 1D Array(array=w2788) -> (reversed array=w2787:T11[])
        n1209 = for {
          tunnel: w2787 -> [w2845] mode=indexing
          tunnel: [w2842] -> w2799 mode=indexing
          tunnel: w2789 -> [w2841]
          tunnel: w2781 -> [w2839]
          n1210 = Unbundle By Name(w2845) -> ("command"=w2844:string, "command data"=w2843:variant)
          n1211 = call "App enquece.vi"("Priority Enquece"=TRUE, "error in (no error)"=w2841, "command data"=w2843, "command"=w2844, "queue in"=w2839) -> ("error out"=w2842:errorcluster)  [unwired: 5 in, 1 out]
        }
        n1212 = Merge Errors(w2802, w2799) -> (w2803:errorcluster)
      }
      frame "Test Channel 6" {
        w2876 = 6  # DUT channel (1-11)
        w2877 = T11 {"command"="", "command data"=variant} ("element")
        n1213 = disable-structure shown="LOGGING==TRUE" {
          disable-tunnel: w2871 -> [w2906 _]
          frame condition #0 (active) {
            n1214 = Empty String/Path?(string/path=w2906) -> (empty?=w2909:bool)
            n1215 = Select(t="Quece timeout", s=w2909, f=w2906) -> (s? t:f=w2905:string)
            n1216 = call "string log (SubVI).vi"("Enum"=enum16{"Init", "Log", "Read"}."Log", "state Name"=w2905) -> ()  [unwired: 8 in, 2 out]
          }
          frame condition #1 {
          }
        }
        n1217 = Build Array("Apps.UI Update", "MEAS.AllRelaysOFF2", "Apps.WaitForEvent") -> (w2853:string[])
        n1218 = for {
          tunnel: [w2896] -> w2861 mode=indexing
          shift-right: [w2897] -> w2863
          shift-left: w2856 -> [w2895]
          tunnel: w2853 -> [w2894] mode=indexing
          n1219 = call "App enquece.vi"("Priority Enquece"=TRUE, "command"=w2894, "queue in"=w2895) -> ("error out"=w2896:errorcluster, "Queue out"=w2897:refnum<queue>)  [unwired: 7 in]
        }
        n1220 = Merge Errors(w2861) -> (w2852:errorcluster)
